vi "Set Voltage by Name.vi"(8 "error in (no error)":errorcluster, 9 "Voltage":dbl format="%#_13g", 10 "Channel_Name":string, 11 "Analog-Output in":refnum<class "Analog-Output.lvclass">) -> (0 "error out":errorcluster, 3 "Analog-Output out":refnum<class "Analog-Output.lvclass">)   [LabVIEW 2019, in "Analog-Output.lvlib" / "Analog-Output.lvclass"]
uses:
  Library/Analog-Output.lvclass
  Library/Analog-Output.lvclass/Analog-Output.ctl
  <vilib>/Utility/error.llb/Error Cluster From Error Code.vi
  <vilib>/ErrorRing/Error Ring.xnode
  builds/Engine/Engine.lvlibp/Project/Engine.lvclass
  C:/Users/Public/Documents/Development/builds/Engine/Engine.lvlibp/Project/Engine.lvclass
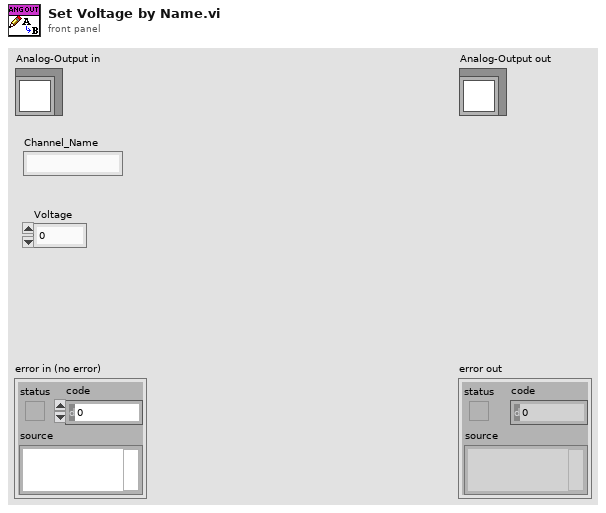
[diagram p1: front panel]
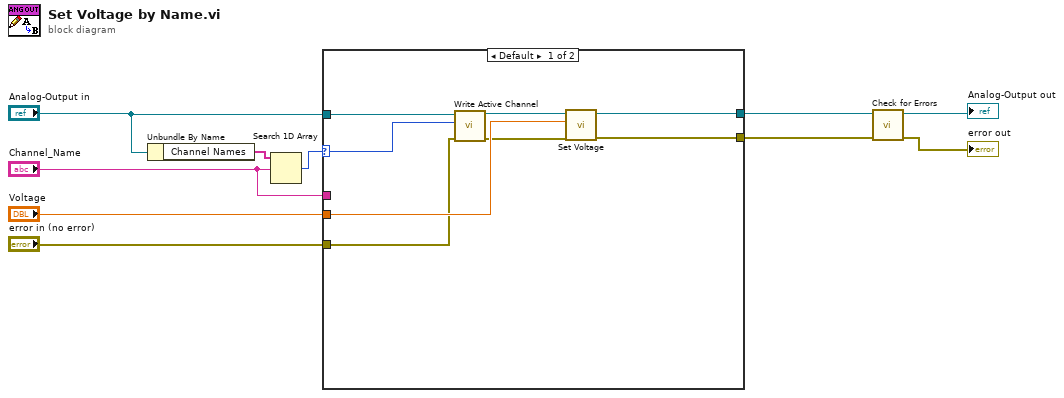
[diagram p0: block diagram]
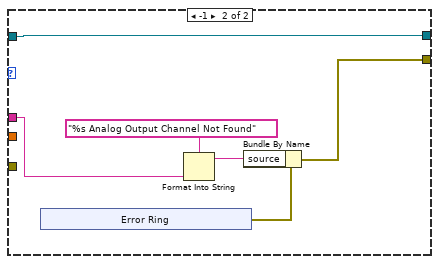
[diagram p2: hidden frame]
diagram:
  n1 = Unbundle By Name("Analog-Output in") -> ("Channel Names"=w4:string[])
  n2 = Search 1D Array(1D array=w4, element="Channel_Name") -> (index of element=w5:i32)  [unwired: 1 in]
  n3 = case shown="Default" w5 {
    selector: w5 -> [w18 _]
    tunnel: "Voltage" -> [w16 _]
    tunnel: "error in (no error)" -> [w13 _]
    tunnel: [w12 w20] -> w6
    tunnel: "Channel_Name" -> [_ w21]
    tunnel: "Analog-Output in" -> [w17 w19]
    tunnel: [w11 w19] -> w2
    frame Default {
      n4 = call "Write Active Channel.vi"("error in (no error)"=w13, "Active Channel"=w18, "Analog-Output in"=w17) -> ("error out"=w14:errorcluster, "Analog-Output out"=w15:refnum<class "Analog-Output.lvclass">)  [unwired: 7 in]
      n5 = call-dynamic "Set Voltage.vi"("error in (no error)"=w14, "Voltage"=w16, "Analog-Output in"=w15) -> ("error out"=w12:errorcluster, "Analog-Output out"=w11:refnum<class "Analog-Output.lvclass">)  [unwired: 7 in]
    }
    frame -1 {
      n6 = xnode "Error Ring"() -> ("error out"=w24:errorcluster)
      n7 = Format Into String(format string="%s Analog Output Channel Not Found" ("source"), w21) -> (resulting string=w22:string)  [unwired: 2 in, 1 out]
      n8 = Bundle By Name(cluster=w24, "source"=w22) -> (w20:errorcluster)
    }
  }
  n9 = call "Check for Errors.vi"("error in"=w6, "Engine in"=w2) -> ("error out"=→"error out":errorcluster, "Engine out"=→"Analog-Output out":refnum<class "Analog-Output.lvclass">)  [unwired: 8 in]
